vi "tcp write.vi"(8 "error in":errorcluster, 9 "termination":string, 10 "Data":string, 11 "Connection in":refnum<k5>) -> (0 "error out":errorcluster)   [LabVIEW 2013]
doc: "# #############################################################################\n# ATTENTION\n# #############################################################################\n#\n# This software is for guidance only. It is provided \"as is\".\n# It only aims at providing coding information to the customer in order for\n# them to save time. As a result no warranties, whether express, implied or\n# statutory, including, but not limited to implied warranties of\n# merchantability and fitness for a particular purpose apply to this software.\n# A·P·E Angewandte Physik und Elektronik GmbH shall not be held liable for any\n# direct, indirect or consequential damages with respect to any claims arising\n# from the content of such sourcecode and/or the use made by customers of the\n# coding information contained herein in connection with their products.\n#\n# #############################################################################"
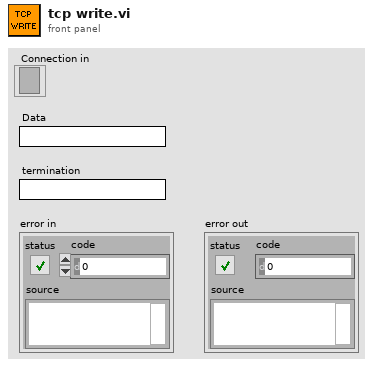
[diagram p1: front panel]
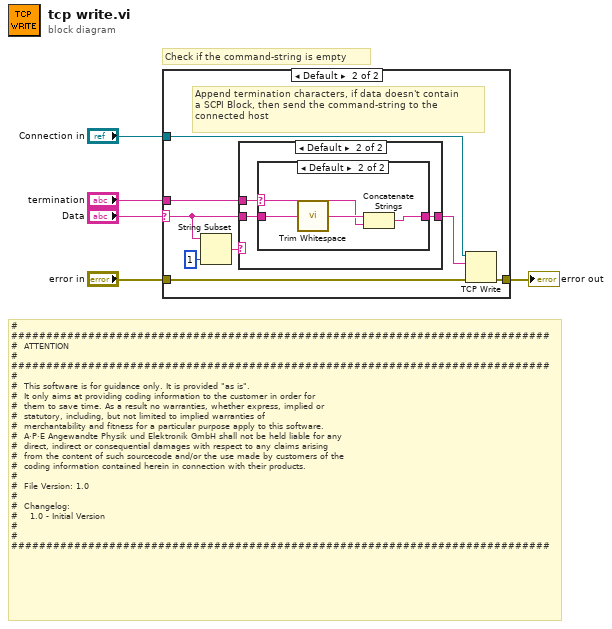
[diagram p0: block diagram]
diagram:
  # "# #############################################################################\n#  ATTENTION\n# #############################################################################\n#\n#  This software is for guidance only. It is provided \"as is\".\n#  It only aims at providing coding information to the customer in order for\n#  them to save time. As a result no warranties, whether express, implied or\n#  statutory, including, but not limited to implied warranties of\n#  merchantability and fitness for a particular purpose apply to this software.\n#  A·P·E Angewandte Physik und Elektronik GmbH shall not be held liable for any\n#  direct, indirect or consequential damages with respect to any claims arising\n#  from the content of such sourcecode and/or the use made by customers of the\n#  coding information contained herein in connection with their products.\n#\n#  File Version: 1.0\n#\n#  Changelog:\n#    1.0 - Initial Version\n#\n# #############################################################################"
  # "Check if the command-string is empty"
  n1 = case shown="Default" "Data" {
    selector: "Data" -> [_ w11]
    tunnel: [w6 w10] -> w4
    tunnel: "error in" -> [w6 w9]
    tunnel: "Connection in" -> [_ w8]
    tunnel: "termination" -> [_ w7]
    frame "" {
    }
    frame Default {
      # "Append termination characters, if data doesn't contain\na SCPI Block, then send the command-string to the \nconnected host"
      n2 = String Subset(string=w11, length (rest)=1 ("length (rest)")) -> (substring=w14:string)  [unwired: 1 in]
      n3 = case shown="Default" w14 {
        tunnel: [w15 w18] -> w12
        tunnel: w11 -> [w15 w17]
        tunnel: w7 -> [_ w16]
        frame "#" {
        }
        frame Default {
          n4 = case shown="Default" w16 {
            selector: w16 -> [_ w20]
            tunnel: [w19 w22] -> w18
            tunnel: w17 -> [w19 w21]
            frame "" {
            }
            frame Default {
              n5 = call <vilib>:"Trim Whitespace.vi"("string"=w21) -> ("trimmed string"=w23:string)  [unwired: 1 in]
              n6 = Concatenate Strings(w23, w20) -> (w22:string)
            }
          }
        }
      }
      n7 = TCP Write(connection ID=w8, data in=w12, error in (no error)=w9) -> (error out=w10:errorcluster)  [unwired: 1 in, 2 out]
    }
  }
  "error out" <- w4
